vi "Register Vecto Services.vi"(8 "error in (no error)":errorcluster, 11 "VolatusCoreTask in":refnum<class "VolatusCoreTask.lvclass">) -> (0 "error out":errorcluster, 3 "VolatusCoreTask out":refnum<class "VolatusCoreTask.lvclass">)   [LabVIEW 2020, in "Volatus.lvlib" / "VolatusCoreTask.lvclass"]
uses:
  VolatusCoreTask.lvclass
  VolatusCoreTask.lvclass/VolatusCoreTask.ctl
  lv-vecto/Vecto/Vecto/Vecto.lvclass
  TelemetryAPI/TelemetryAPI.lvclass
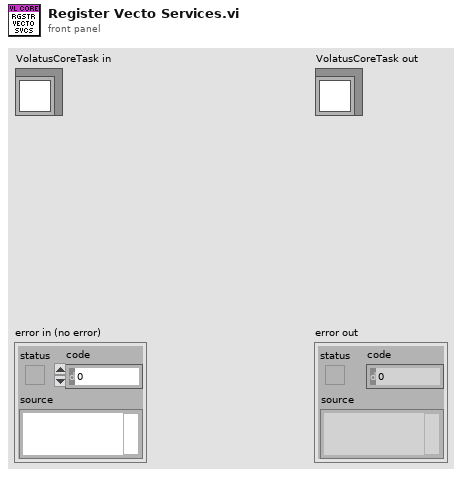
[diagram p1: front panel]
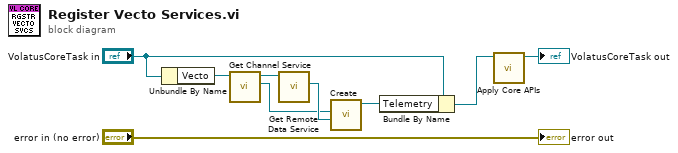
[diagram p0: block diagram]
diagram:
  n1 = Unbundle By Name("VolatusCoreTask in") -> ("Vecto"=w8:refnum<class "Vecto.lvclass">)
  n2 = call "Get Channel Service.vi"("Vecto in"=w8) -> ("ChannelService"=w5:refnum<class "ChannelService.lvclass">, "Vecto out"=w7:refnum<class "Vecto.lvclass">)  [unwired: 8 in, 1 out]
  n3 = call "Get Remote Data Service.vi"("Vecto in"=w7) -> ("RemoteDataService"=w6:refnum<class "RemoteDataService.lvclass">)  [unwired: 8 in, 2 out]
  n4 = call "Create.vi"("RemoteDataService"=w6, "ChannelService"=w5) -> ("TelemetryAPI out"=w4:refnum<class "TelemetryAPI.lvclass">)  [unwired: 8 in, 1 out]
  n5 = Bundle By Name(cluster="VolatusCoreTask in", "Telemetry"=w4) -> (w2:refnum<class "VolatusCoreTask.lvclass">)
  n6 = call "Apply Core APIs.vi"("VolatusCoreTask in"=w2) -> ("VolatusCoreTask out"=→"VolatusCoreTask out":refnum<class "VolatusCoreTask.lvclass">)  [unwired: 9 in, 1 out]
  "error out" <- "error in (no error)"
